vi "CAL-SPL to V Interp.vi"(0 "user path":path, 7 "Fi (Hz)":dbl[](array[numeric]), 11 "dB SPL":dbl) -> (4 "Amplitude (V)":dbl[](array[numeric]), 8 "Phase (cycles)":dbl[](array[numeric]))   [LabVIEW 2020]
uses:
  epl-vi-lib/Utility VIs/Math VIs/dB to Linear (1D).vi
  epl-vi-lib/Utility VIs/Math VIs/Linear to dB (array).vi
  epl-vi-lib/Utility VIs/Math VIs/dB to Linear (scalar).vi
  <vilib>/gmath/NI_Gmath.lvlib
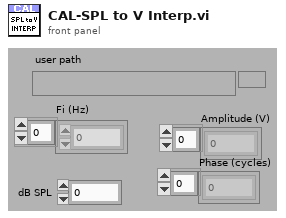
[diagram p1: front panel]
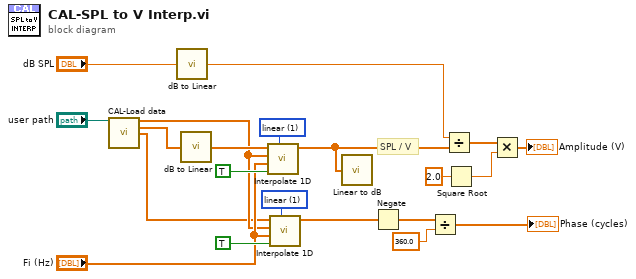
[diagram p0: block diagram]
diagram:
  w19 = 1 items=["nearest", "linear", "spline", "cubic Hermite", "Lagrange"] ("method")
  w21 = 1 items=["nearest", "linear", "spline", "cubic Hermite", "Lagrange"] ("method")
  # "SPL / V"
  n1 = call "CAL-Load data.vi"("user path"="user path") -> ("Frequency (Hz)"=w15:dbl[], "Mag"=w14:dbl[], "Phase"=w13:dbl[])  [unwired: 7 in, 5 out]
  n2 = call-poly "dB to Linear.vi"("dB"="dB SPL") -> ("linear"=w10:dbl)
  n3 = call-poly "dB to Linear.vi"("dB"=w14) -> ("linear"=w17:dbl[])
  n4 = call <vilib>:"Interpolate 1D.vi"("method"=w21, "X is monotonic"=TRUE, "xi"="Fi (Hz)", "X"=w15, "Y"=w17) -> ("yi"=w1:dbl[])  [unwired: 4 in, 2 out]
  n5 = call <vilib>:"Interpolate 1D.vi"("method"=w19, "X is monotonic"=TRUE, "xi"="Fi (Hz)", "X"=w15, "Y"=w13) -> ("yi"=w8:dbl[])  [unwired: 4 in, 2 out]
  n6 = call-poly "Linear to dB.vi"("linear"=w1) -> ()  [unwired: 1 out]
  n7 = Negate(x=w8) -> (-x=w7:dbl[])
  n8 = Divide(x=w7, y=360.0) -> (x/y=→"Phase (cycles)":dbl[])
  n9 = Divide(x=w10, y=w1) -> (x/y=w9:dbl[])
  n10 = Square Root(x=2.0) -> (sqrt(x)=w4:dbl)
  n11 = Multiply(x=w9, y=w4) -> (x*y=→"Amplitude (V)":dbl[])
